vi "initialize vi references.vi"(7 "runtime class path":path, 8 "error in":errorcluster, 9 "output in":T4, 10 "process in":T5, 11 "input in":T3) -> (0 "error out":errorcluster, 3 "initialized references":T1[](array[typedef]))   [LabVIEW 2013]
uses:
  Controls/processing script control.ctl
  Controls/output script control.ctl
  Controls/input script control.ctl
  Controls/initialized references.ctl
  Controls/interface VI type.ctl
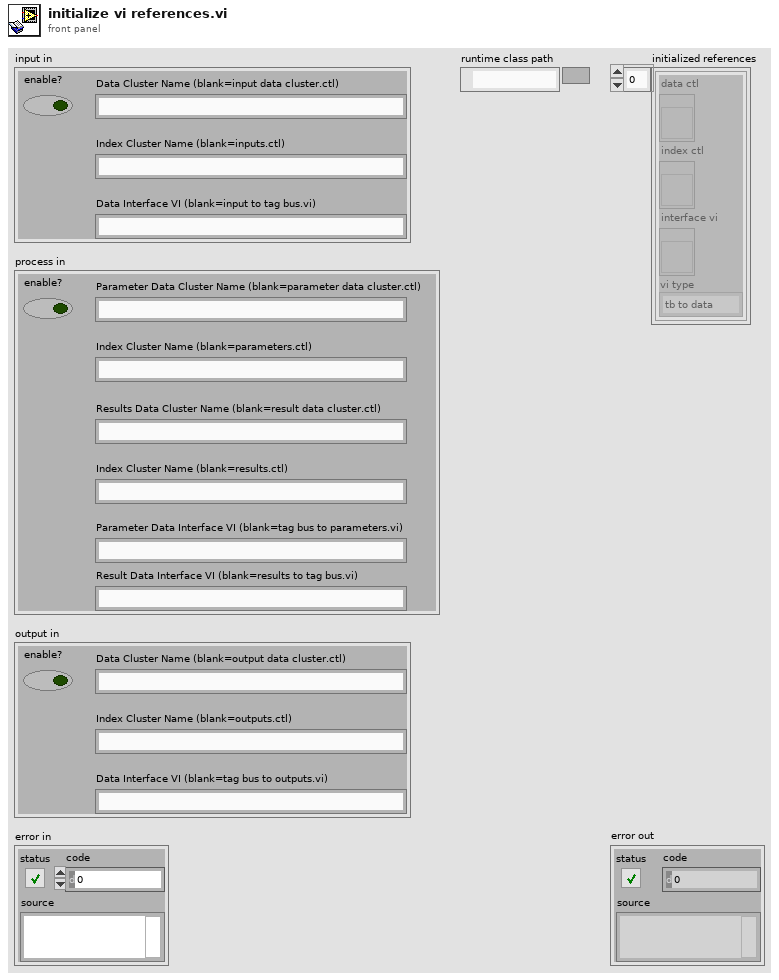
[diagram p1: front panel]
types:
  T1 = typedef "initialized references.ctl" = cluster{"data ctl":refnum<vi>, "index ctl":refnum<vi>, "interface vi":refnum<vi>, "vi type":T2}
  T2 = typedef "interface VI type.ctl" = enum16{"tb to data", "data to tb"}
  T3 = typedef "input script control.ctl" = cluster{"enable?":bool, "Data Cluster Name (blank=input data cluster.ctl)":string, "Index Cluster Name (blank=inputs.ctl)":string, "Data Interface VI (blank=input to tag bus.vi)":string}
  T4 = typedef "output script control.ctl" = cluster{"enable?":bool, "Data Cluster Name (blank=output data cluster.ctl)":string, "Index Cluster Name (blank=outputs.ctl)":string, "Data Interface VI (blank=tag bus to outputs.vi)":string}
  T5 = typedef "processing script control.ctl" = cluster{"enable?":bool, "Parameter Data Cluster Name (blank=parameter data cluster.ctl)":string, "Index Cluster Name (blank=parameters.ctl)":string, "Results Data Cluster Name (blank=result data cluster.ctl)":string, "Index Cluster Name (blank=results.ctl)":string, "Parameter Data Interface VI (blank=tag bus to parameters.vi)":string, "Result Data Interface VI (blank=results to tag bus.vi)":string}
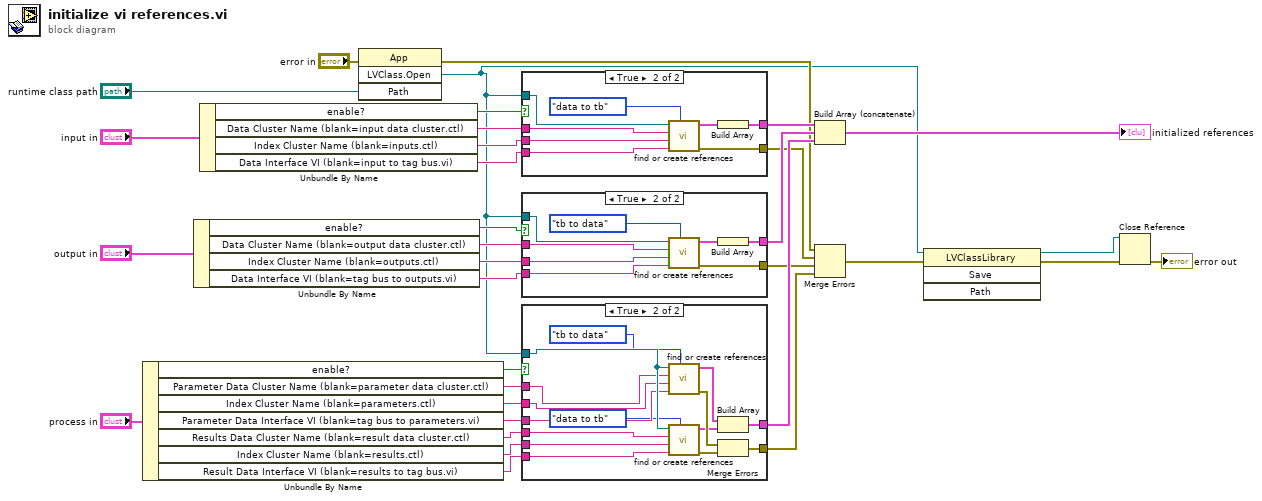
[diagram p0: block diagram]
diagram:
  n1 = Unbundle By Name("process in") -> ("enable?"=w24:bool, "Parameter Data Cluster Name (blank=parameter data cluster.ctl)"=w23:string, "Index Cluster Name (blank=parameters.ctl)"=w22:string, "Parameter Data Interface VI (blank=tag bus to parameters.vi)"=w21:string, "Results Data Cluster Name (blank=result data cluster.ctl)"=w16:string, "Index Cluster Name (blank=results.ctl)"=w17:string, "Result Data Interface VI (blank=results to tag bus.vi)"=w18:string)
  n2 = Unbundle By Name("output in") -> ("enable?"=w25:bool, "Data Cluster Name (blank=output data cluster.ctl)"=w26:string, "Index Cluster Name (blank=outputs.ctl)"=w27:string, "Data Interface VI (blank=tag bus to outputs.vi)"=w28:string)
  n3 = Unbundle By Name("input in") -> ("enable?"=w32:bool, "Data Cluster Name (blank=input data cluster.ctl)"=w31:string, "Index Cluster Name (blank=inputs.ctl)"=w30:string, "Data Interface VI (blank=input to tag bus.vi)"=w29:string)
  n4 = invoke class="App" method="LVClass.Open"(error in="error in", "Path"="runtime class path") -> (error out=w5:errorcluster, "LVClass.Open"=w2:refnum<vi>)  [unwired: 2 in, 2 out]
  n5 = case shown="True" w32 {
    tunnel: w31 -> [_ w41]
    tunnel: w30 -> [_ w39]
    tunnel: w29 -> [_ w38]
    tunnel: w2 -> [_ w40]
    tunnel: [_ w36] -> w14
    tunnel: [_ w35] -> w7
    frame False {
    }
    frame True {
      n6 = call "find or create references.vi"("vi type"=interface_VI_type."data to tb", "Data Interface VI"=w38, "Index Cluster Name"=w39, "Data Cluster Name"=w41, "LVClassLibrary in"=w40) -> ("error out"=w35:errorcluster, "vi refs"=w37:T1)  [unwired: 5 in]
      n7 = Build Array(w37) -> (w36:T1[])
    }
  }
  n8 = case shown="True" w25 {
    tunnel: w26 -> [_ w46]
    tunnel: w27 -> [_ w45]
    tunnel: w28 -> [_ w44]
    tunnel: [_ w48] -> w13
    tunnel: w2 -> [_ w47]
    tunnel: [_ w43] -> w6
    frame False {
    }
    frame True {
      n9 = call "find or create references.vi"("vi type"=interface_VI_type."tb to data", "Data Interface VI"=w44, "Index Cluster Name"=w45, "Data Cluster Name"=w46, "LVClassLibrary in"=w47) -> ("error out"=w43:errorcluster, "vi refs"=w49:T1)  [unwired: 5 in]
      n10 = Build Array(w49) -> (w48:T1[])
    }
  }
  n11 = case shown="True" w24 {
    tunnel: w23 -> [_ w52]
    tunnel: w22 -> [_ w53]
    tunnel: w21 -> [_ w54]
    tunnel: w18 -> [_ w57]
    tunnel: w17 -> [_ w56]
    tunnel: w16 -> [_ w55]
    tunnel: [_ w63] -> w10
    tunnel: [_ w59] -> w8
    tunnel: w2 -> [_ w58]
    frame False {
    }
    frame True {
      n12 = call "find or create references.vi"("vi type"=interface_VI_type."tb to data", "Data Interface VI"=w54, "Index Cluster Name"=w53, "Data Cluster Name"=w52, "LVClassLibrary in"=w58) -> ("error out"=w62:errorcluster, "vi refs"=w64:T1)  [unwired: 5 in]
      n13 = call "find or create references.vi"("vi type"=interface_VI_type."data to tb", "Data Interface VI"=w57, "Index Cluster Name"=w56, "Data Cluster Name"=w55, "LVClassLibrary in"=w58) -> ("error out"=w61:errorcluster, "vi refs"=w60:T1)  [unwired: 5 in]
      n14 = Build Array(w64, w60) -> (w63:T1[])
      n15 = Merge Errors(w62, w61) -> (w59:errorcluster)
    }
  }
  n16 = Build Array (concatenate)(w14, w13, w10) -> (→"initialized references":T1[])
  n17 = Merge Errors(w5, w7, w6, w8) -> (w11:errorcluster)
  n18 = invoke class="LVClassLibrary" method="Save"(reference=w2, error in=w11) -> (reference out=w1:refnum<vi>, error out=w3:errorcluster)  [unwired: 2 in, 2 out]
  n19 = Close Reference(reference=w1, error in (no error)=w3) -> (error out=→"error out":errorcluster)
